vi "Pre Launch Init.vi"(11 "Debug Monitor in":refnum<class "Debug Monitor.lvclass">) -> (0 "error out":errorcluster, 3 "Debug Monitor out":refnum<class "Debug Monitor.lvclass">)   [LabVIEW 2017, in "Debug Monitor.lvclass"]
doc: "(<B>Filename</B>: Actor Framework.lvlib:Actor.lvclass:Pre Launch Init.vi)\n\nDefines behavior that occurs after the Launch Nested Actor method is invoked but before the actor's Actor Core method begins running.\n\nBy default, this method does nothing. A descendant class may override it to define behavior."
uses:
  Debug Monitor.lvclass
  Source/Monitor Data/Monitor Data.lvclass
  Debug Monitor.lvclass/Debug Monitor.ctl
  Source/Actor Monitor/Actor Monitor/Actor Monitor.lvclass
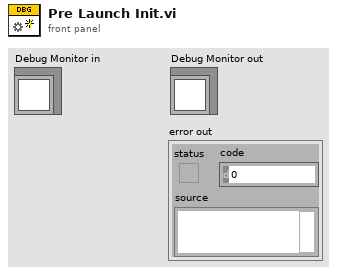
[diagram p1: front panel]
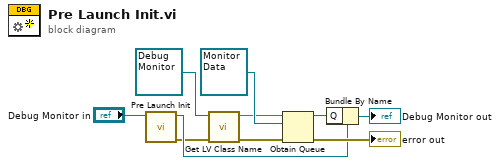
[diagram p0: block diagram]
diagram:
  n1 = call-parent "Pre Launch Init.vi"("Actor in"="Debug Monitor in") -> ("error out"=w4:errorcluster, "Actor out"=w5:refnum<class "Debug Monitor.lvclass">)  [unwired: 9 in]
  n2 = call <vilib>:"Get LV Class Name.vi"("error in (no error)"=w4, "object"=refnum<class "Debug Monitor.lvclass"> refnum ("Actor out")) -> ("error out"=w2:errorcluster, "class name"=w3:string)  [unwired: 8 in]
  n3 = Obtain Queue(name (unnamed)=w3, element data type=refnum<class "Monitor Data.lvclass"> refnum ("Monitor Data"), error in (no error)=w2) -> (queue out=w7:refnum<queue>, error out=→"error out":errorcluster)  [unwired: 2 in, 1 out]
  n4 = Bundle By Name(cluster=w5, "Q"=w7) -> (→"Debug Monitor out":refnum<class "Debug Monitor.lvclass">)
